vi "Get VI Info.vi"(1 "vi path":path=path "C:/Users/zhyang/Desktop/VIAnalyser/Rename Chassis and All Connected Modules(Template).vi") -> (0 "temporary HTML file created":path)   [LabVIEW 2016]
uses:
  <vilib>/Utility/NIReport.llb/image depth.ctl
  <vilib>/Utility/NIReport.llb/Append Report Text (str wrap).vi
  <vilib>/printing/OpenHTMLReport.llb/Open HTML Report in Browser (Refnum).vi
  <vilib>/Utility/NIReport.llb/NI_report.lvclass
  <vilib>/Utility/NIReport.llb/NI_ReportGenerationCore.lvlib
panel:
  out "error out 2":errorcluster
  out "pane view":picture
  in  "picture":picture
  out "Automatic Error Handling":bool
  out "Execution:Priority":T1(ring)
  out "Execution:Preferred Exec System":T2(ring)
  out "Execution:Inline SubVI":bool
  out "Execution:Allow Debugging":bool
  out "error out":errorcluster
  out "VI Description":string
  out "VI Name":string
  out "VI Path":path
  out "Execution:Is Reentrant":bool
  out "VI Type":T3(ring)
  out "Execution:Reentrancy Type":T4(ring)
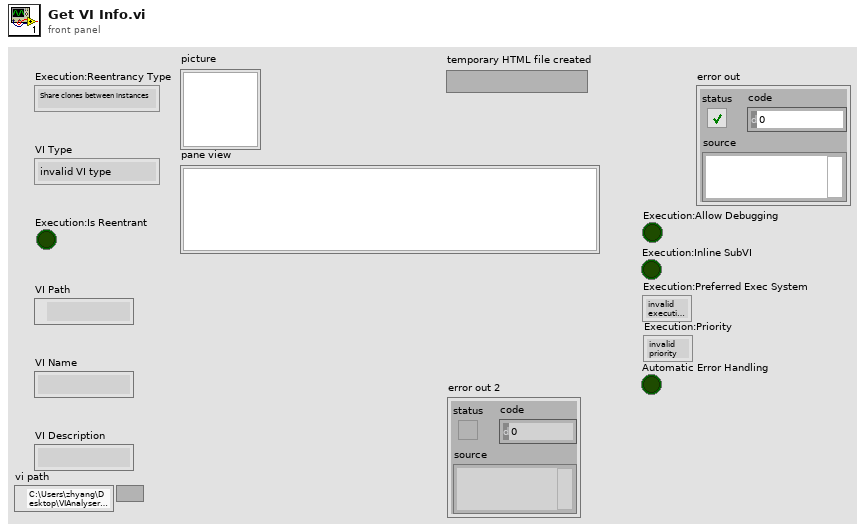
[diagram p1: front panel]
types:
  T1 = enum32{"invalid priority", "background priority", "normal priority", "above normal priority", "high priority", "time critical priority", "subroutine"}
  T2 = enum32{"invalid execution system", "user interface", "standard", "instrument i/o", "data acquisition", "other 1", "other 2", "same as caller"}
  T3 = enum32{"invalid VI type", "Standard VI", "Control VI", "Global VI", "Polymorphic VI", "Configuration VI", "SubSystem", "Facade VI", "Method VI", "Statechart Diagram VI"}
  T4 = enum16{"Share clones between instances", "Preallocate clone for each instance"}
  T5 = typedef "NI_ReportGenerationCore.lvlib/image depth.ctl" = u16
  T6 = enum16{"Standard Report", "HTML", "Word", "Excel"}
  T7 = typedef "imagedata.ctl" = cluster{"image type":i32, "image depth":i32, "image":u8[], "mask":u8[], "colors":u32[], "Rectangle":cluster{"left":i16, "top":i16, "right":i16, "bottom":i16}}
  T8 = enum16{"Invalid Wire Rule", "Required", "Recommended", "Optional", "Dynamic Dispatch"}[]
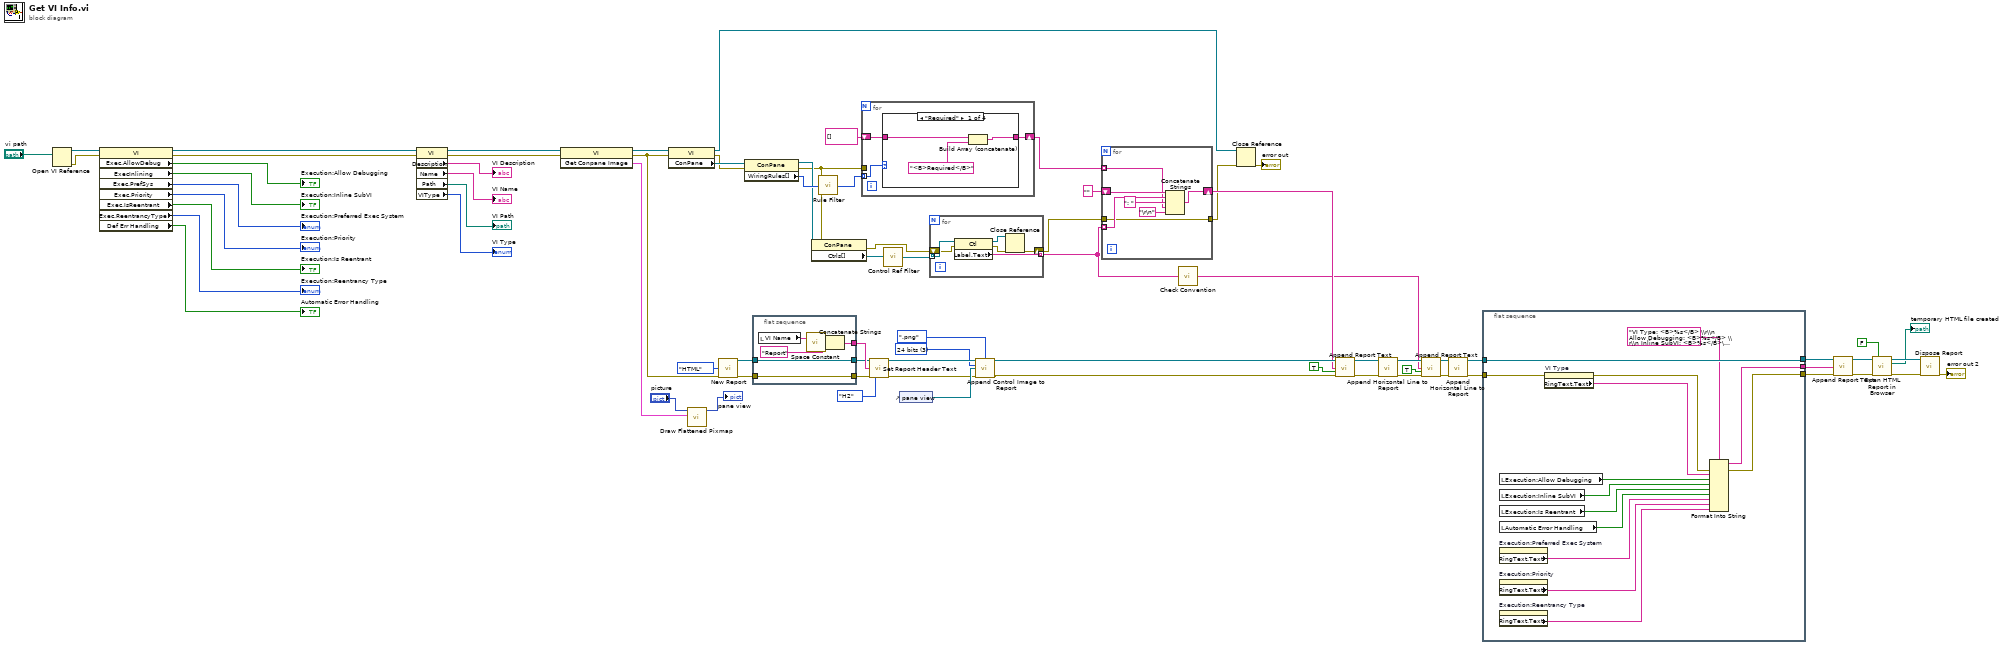
[diagram p0: block diagram]
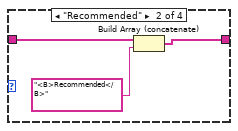
[diagram p2: hidden frame]
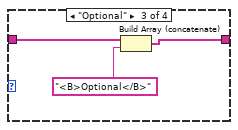
[diagram p3: hidden frame]
diagram:
  w51 = T5 3 items=["B&W", "4 bits", "8 bits", "24 bits"] ("image depth")
  n1 = Open VI Reference(vi path="vi path") -> (vi reference=w73:refnum<vi>, error out=w58:errorcluster)  [unwired: 5 in]
  n2 = property class="VI"(reference=w73, error in=w58) -> (reference out=w72:refnum<vi>, error out=w71:errorcluster, "Exec.AllowDebug"=→"Execution:Allow Debugging":bool, "ExecInlining"=→"Execution:Inline SubVI":bool, "Exec.PrefSys"=→"Execution:Preferred Exec System":T2, "Exec.Priority"=→"Execution:Priority":T1, "Exec.IsReentrant"=→"Execution:Is Reentrant":bool, "Exec.ReentrancyType"=→"Execution:Reentrancy Type":T4, "Def Err Handling"=→"Automatic Error Handling":bool)
  n3 = property class="VI"(reference=w72, error in=w71) -> (reference out=w70:refnum<vi>, error out=w69:errorcluster, "Description"=→"VI Description":string, "Name"=→"VI Name":string, "Path"=→"VI Path":path, "VIType"=→"VI Type":T3)
  n4 = invoke class="VI" method="Get Conpane Image"(reference=w70, error in=w69) -> (reference out=w42:refnum<vi>, error out=w41:errorcluster, "Get Conpane Image"=w55:T7)  [unwired: 1 in]
  n5 = property class="VI"(reference=w42, error in=w41) -> (reference out=w31:refnum<vi>, error out=w39:errorcluster, "ConPane"=w40:refnum<vi>)
  n6 = call <vilib>:"Draw Flattened Pixmap.vi"("image data"=w55, "picture"="picture") -> ("new picture"=→"pane view":picture)  [unwired: 7 in]
  n7 = call <vilib>:"New Report.vi"("report type"=T6."HTML", "error in (no error)"=w41) -> ("report out"=w11:refnum<class "NI_report.lvclass">, "error out"=w13:errorcluster)  [unwired: 12 in]
  n8 = property class="ConPane"(reference=w40, error in=w39) -> (reference out=w7:refnum<vi>, error out=w6:errorcluster, "WiringRules[]"=w9:T8)
  n9 = flat-sequence {
    tunnel: [w80] -> w15
    tunnel: w13 -> [w77]
    tunnel: [w77] -> w12
    tunnel: w11 -> [w76]
    tunnel: [w76] -> w10
    frame #0 {
      n10 = local read "VI Name"() -> (w81:string)
      n11 = call <vilib>:"Space Constant.vi"() -> ("String"=w79:string)
      n12 = Concatenate Strings(w81, w79, "Report" ("string")) -> (w80:string)
    }
  }
  n13 = property class="ConPane"(reference=w7, error in=w6) -> (error out=w3:errorcluster, "Ctrls[]"=w5:refnum<vi>[])  [unwired: 1 out]
  n14 = call "Rule Filter.vi"("WiringRules[]"=w9) -> ("wiring rules"=w8:T8)
  n15 = for {
    tunnel: w6 -> [_]
    tunnel: w8 -> [w84] mode=indexing
    shift-right: [w82] -> w32
    shift-left: string[] [] -> [w83]
    n16 = case shown="\"Required\"" w84 {
      tunnel: w83 -> [w87 w90 w93 w94]
      tunnel: [w85 w88 w91 w94] -> w82
      frame "Required" {
        n17 = Build Array (concatenate)(w87, "<B>Required</B>") -> (w85:string[])
      }
      frame "Recommended" {
        n18 = Build Array (concatenate)(w90, "<B>Recommended</B>") -> (w88:string[])
      }
      frame "Optional" {
        n19 = Build Array (concatenate)(w93, "<B>Optional</B>") -> (w91:string[])
      }
      frame Default {
      }
    }
  }
  n20 = call-dynamic "Set Report Header Text.vi"("report in"=w10, "center header text"=w15, "error in (no error)"=w12, "HTML header size"=enum16{"H1", "H2", "H3", "H4", "H5", "H6", "H7"}."H2") -> ("report out"=w52:refnum<class "NI_report.lvclass">, "error out"=w47:errorcluster)  [unwired: 10 in]
  n21 = call "Control Ref Filter.vi"("Controls[]"=w5) -> ("valide controls"=w4:refnum<vi>[])
  n22 = control-ref of="pane view"() -> (w48:refnum<vi>)
  n23 = for {
    tunnel: w4 -> [w100] mode=indexing
    tunnel: [w99] -> w2 mode=indexing
    shift-right: [w95] -> w1
    shift-left: w3 -> [w98]
    n24 = property class="Ctl"(reference=w100, error in=w98) -> (reference out=w96:refnum<vi>, error out=w97:errorcluster, "Label.Text"=w99:string)
    n25 = Close Reference(reference=w96, error in (no error)=w97) -> (error out=w95:errorcluster)
  }
  n26 = call-dynamic "Append Control Image to Report.vi"("report in"=w52, "image file type (.jpg)"=enum16{".jpg", ".png"}.".png" ("image file type"), "image depth"=w51, "ctrl reference"=w48, "error in (no error)"=w47) -> ("report out"=w43:refnum<class "NI_report.lvclass">, "error out"=w25:errorcluster)  [unwired: 7 in, 2 out]
  n27 = for {
    tunnel: w2 -> [w106] mode=indexing
    tunnel: w32 -> [w104] mode=indexing
    tunnel: w1 -> [w101]
    shift-right: [w102] -> w37
    shift-left: "" -> [w107]
    tunnel: [w101] -> w34
    n28 = Concatenate Strings(w107, w106, ": " ("string"), w104, "\r\n") -> (w102:string)
  }
  n29 = call "Check Convention.vi"("terminal name array"=w2) -> ("validation result"=w28:string)
  n30 = Close Reference(reference=w31, error in (no error)=w34) -> (error out=→"error out":errorcluster)
  n31 = call-poly <vilib>:"Append Report Text.vi"("report in"=w43, "text"=w37, "append on new line? (F)"=TRUE, "error in (no error)"=w25) -> ("report out"=w45:refnum<class "NI_report.lvclass">, "error out"=w44:errorcluster)  [unwired: 8 in, 2 out]
  n32 = call-dynamic "Append Horizontal Line to Report.vi"("report in"=w45, "error in (no error)"=w44) -> ("report out"=w36:refnum<class "NI_report.lvclass">, "error out"=w29:errorcluster)  [unwired: 12 in]
  n33 = call-poly <vilib>:"Append Report Text.vi"("report in"=w36, "text"=w28, "append on new line? (F)"=TRUE, "error in (no error)"=w29) -> ("report out"=w30:refnum<class "NI_report.lvclass">, "error out"=w22:errorcluster)  [unwired: 8 in, 2 out]
  n34 = call-dynamic "Append Horizontal Line to Report.vi"("report in"=w30, "error in (no error)"=w22) -> ("report out"=w20:refnum<class "NI_report.lvclass">, "error out"=w21:errorcluster)  [unwired: 12 in]
  n35 = flat-sequence {
    tunnel: [w118] -> w24
    tunnel: [w116] -> w23
    tunnel: w21 -> [w121]
    tunnel: w20 -> [w118]
    tunnel: [w115] -> w18
    frame #0 {
      n36 = local read "Execution:Allow Debugging"() -> (w119:bool)
      n37 = local read "Execution:Inline SubVI"() -> (w114:bool)
      n38 = local read "Execution:Is Reentrant"() -> (w112:bool)
      n39 = local read "Automatic Error Handling"() -> (w111:bool)
      n40 = property on="Execution:Preferred Exec System" class="Enum (strict)"() -> ("RingText.Text"=w110:string)  [unwired: 2 in, 2 out]
      n41 = property on="Execution:Priority" class="Enum (strict)"() -> ("RingText.Text"=w109:string)  [unwired: 2 in, 2 out]
      n42 = property on="Execution:Reentrancy Type" class="Enum (strict)"() -> ("RingText.Text"=w108:string)  [unwired: 2 in, 2 out]
      n43 = property on="VI Type" class="Enum (strict)"(error in=w121) -> (error out=w117:errorcluster, "RingText.Text"=w120:string)  [unwired: 1 in, 1 out]
      n44 = Format Into String(format string="VI Type: <B>%s</B> \\r\\n Allow Debugging: <B>%s</B> \\r\\n Inline SubVI: <B>%s</B>\\r\\n Is Reentrant: <B>%s</B> \\r\\n Automatic Error Handling: <B>%s</B> \\r\\n Preferred Exec System: <B>%s</B> \\r\\nPriority: <B>%s</B> \\r\\n Reentrancy Type: <B>%s</B> \\r\\n ", error in=w117, w120, w119, w114, w112, w111, w110, w109, w108) -> (resulting string=w115:string, error out=w116:errorcluster)  [unwired: 1 in]
    }
  }
  n45 = call-poly <vilib>:"Append Report Text.vi"("report in"=w24, "text"=w18) -> ("report out"=w19:refnum<class "NI_report.lvclass">)  [unwired: 10 in, 3 out]
  n46 = call-poly <vilib>:"Open HTML Report in Browser.vi"("report in"=w19, "Open in browser?"=FALSE, "error in (no error)"=w23) -> ("report out"=w35:refnum<class "NI_report.lvclass">, "temporary HTML file created"=→"temporary HTML file created":path, "error out"=w26:errorcluster)  [unwired: 10 in]
  n47 = call-dynamic "Dispose Report.vi"("report in"=w35, "error in (no error)"=w26) -> ("error out"=→"error out 2":errorcluster)  [unwired: 13 in]
